vi "Saving shit.vi"() -> ()   [LabVIEW 2009]
panel:
  in  "Unsorted Waypoints":cluster{"Longitude":dbl, "Latitude":dbl}[](array[cluster])
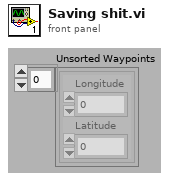
[diagram p1: front panel]
types:
  T1 = enum16{"open", "replace", "create", "open or create", "replace or create", "replace or create with confirmation"}
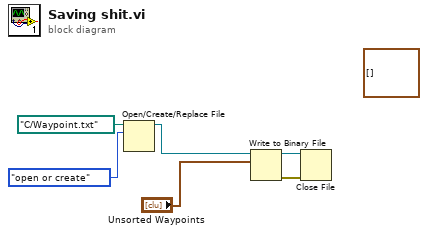
[diagram p0: block diagram]
diagram:
  (unwired) cluster{"Longitude":dbl, "Latitude":dbl}[] [] ("Unsorted Waypoints")
  n1 = Open/Create/Replace File(file path (use dialog)=path "C:/Waypoint.txt", operation (0:open)=T1."open or create") -> (refnum out=w2:refnum<file>)  [unwired: 4 in, 2 out]
  n2 = Write to Binary File(file (use dialog)=w2, data="Unsorted Waypoints") -> (refnum out=w4:refnum<file>, error out=w3:errorcluster)  [unwired: 4 in, 1 out]
  n3 = Close File(refnum=w4, error in=w3) -> ()  [unwired: 2 out]
